vi "Cleanup.vi"(8 "error in (no error)":errorcluster, 11 "Element A in":refnum<class "Element B.lvclass">) -> (0 "error out":errorcluster)   [LabVIEW 2018, in "Array Example.lvlib" / "Element B.lvclass"]
uses:
  Element B.lvclass
  Element Base/Element Base.lvclass
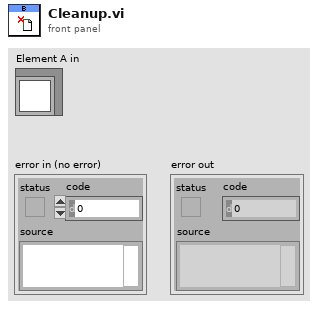
[diagram p1: front panel]
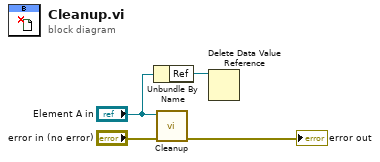
[diagram p0: block diagram]
diagram:
  n1 = Unbundle By Name("Element A in") -> ("Ref"=w4:refnum<data-value>)
  n2 = call-parent "Cleanup.vi"("error in (no error)"="error in (no error)", "ArrayPanel in"="Element A in") -> ("error out"=→"error out":errorcluster)  [unwired: 9 in]
  n3 = Delete Data Value Reference(data value reference=w4) -> ()  [unwired: 1 in, 2 out]
